vi "Markov Estimation.vi"(3 "UDP error in":errorcluster, 4 "UDP input cluster":T4, 5 "USRP error in":errorcluster, 6 "USRP input cluster":T3) -> (0 "ERROR":bool, 1 "UDP output cluster":T2, 2 "USRP output cluster":T1)   [LabVIEW 2014]
panel:
  out "Power":dbl[][](array[numeric])
  out "Delay":dbl[][](array[numeric])
  in  "Tab":enum32{"Interference", "Delay"}(tab)
  out "USRP error":errorcluster
  in  "Sampling Para.":T5={"Method"=enum."Binary", "offset"=0, "threshold"=1.0, "step"=1.0}
  in  "Number of Samplings":i32=100
  out "UDP error":errorcluster
  in  "Sampling Para2":T5
  in  "UDP parameter":T6={"remote IP Address"="192.168.1.101", "remote port"=54322, "local port(Tx)"=54321, "local port(Rx)"=54323}
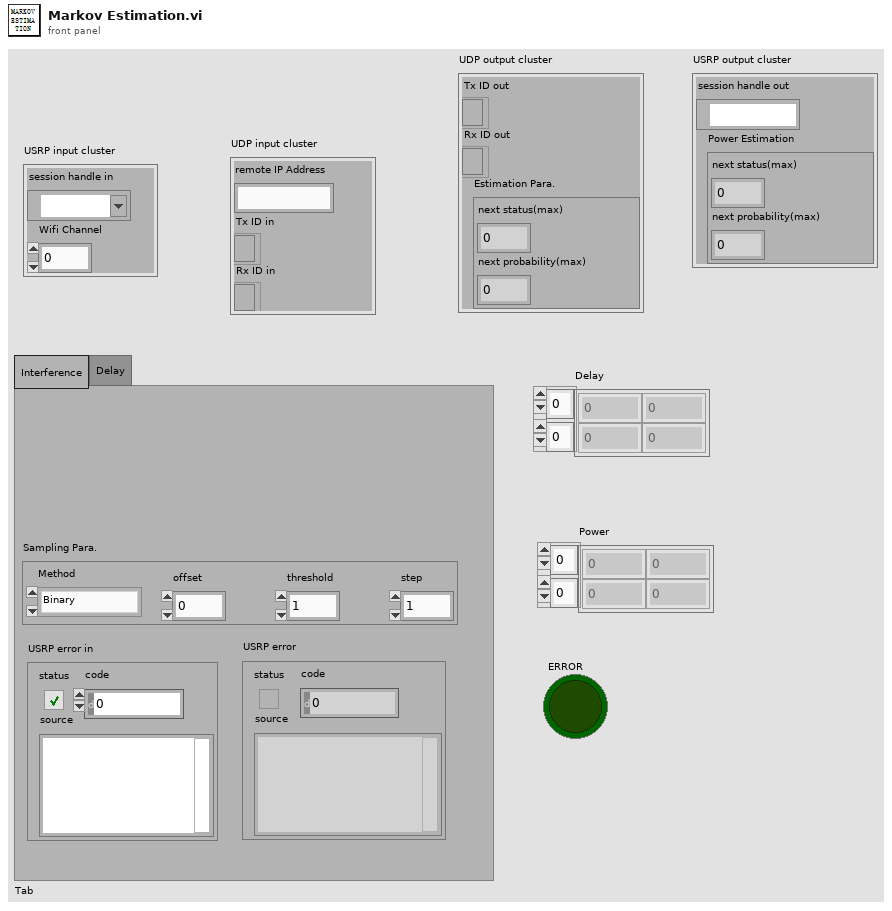
[diagram p1: front panel]
types:
  T1 = cluster{"session handle out":refnum<k15>, "Power Estimation":cluster{"next status(max)":i32, "next probability(max)":dbl}}
  T2 = cluster{"Tx ID out":refnum<k16>, "Rx ID out":refnum<k16>, "Estimation Para.":cluster{"next status(max)":i32, "next probability(max)":dbl}}
  T3 = cluster{"session handle in":refnum<k15>, "Wifi Channel":i32}
  T4 = cluster{"remote IP Address":string, "Tx ID in":refnum<k16>, "Rx ID in":refnum<k16>}
  T5 = cluster{"Method":enum16{"Binary", "Uniform"}, "offset":i32, "threshold":dbl, "step":dbl}
  T6 = cluster{"remote IP Address":string, "remote port":u16, "local port(Tx)":u16, "local port(Rx)":u16}
  T7 = cluster{"Tx ID out":refnum<k16>, "Rx ID out":refnum<k16>, "Delay Estimation":cluster{"next status(max)":i32, "next probability(max)":dbl}}
  T8 = cluster{"next status(max)":i32, "next probability(max)":dbl}
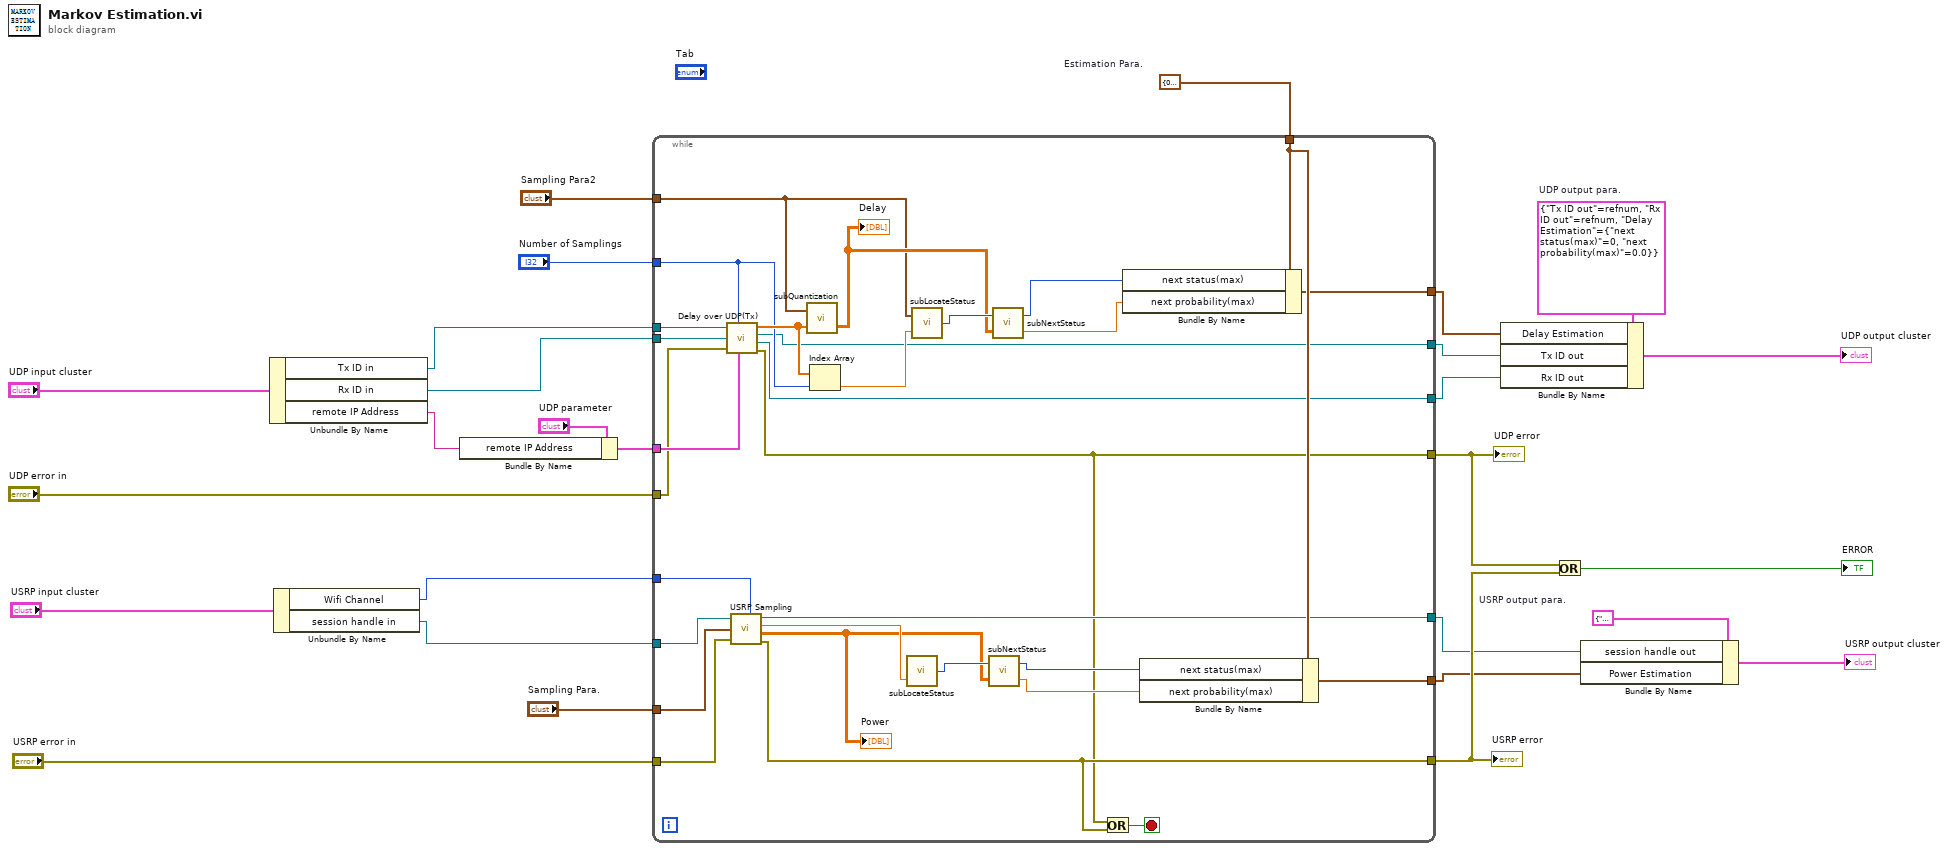
[diagram p0: block diagram]
diagram:
  w4 = T1 {"session handle out"="", "Power Estimation"={"next status(max)"=0, "next probability(max)"=0.0}}  # USRP output para.
  w9 = T7 {"Tx ID out"=refnum, "Rx ID out"=refnum, "Delay Estimation"={"next status(max)"=0, "next probability(max)"=0.0}}  # UDP output para.
  w24 = T8 {"next status(max)"=0, "next probability(max)"=0.0}  # Estimation Para.
  n1 = Unbundle By Name("UDP input cluster") -> ("Tx ID in"=w15:refnum<k16>, "Rx ID in"=w14:refnum<k16>, "remote IP Address"=w13:string)
  n2 = Unbundle By Name("USRP input cluster") -> ("Wifi Channel"=w11:i32, "session handle in"=w10:refnum<k15>)
  n3 = Bundle By Name(cluster="UDP parameter", "remote IP Address"=w13) -> (w17:T6)
  n4 = while {
    tunnel: [w56] -> w26
    tunnel: "Sampling Para2" -> [w50]
    tunnel: w24 -> [w49]
    tunnel: [w44] -> w8
    tunnel: [w43] -> w2
    tunnel: [w42] -> w3
    tunnel: "USRP error in" -> [w41]
    tunnel: w10 -> [w40]
    tunnel: "Sampling Para." -> [w39]
    tunnel: w11 -> [w38]
    tunnel: w17 -> [w37]
    tunnel: "UDP error in" -> [w36]
    tunnel: "Number of Samplings" -> [w33]
    tunnel: [w28] -> w19
    tunnel: w15 -> [w32]
    tunnel: w14 -> [w31]
    tunnel: [w30] -> w7
    tunnel: [w29] -> w6
    stop <- w57 stop-if-true
    n5 = call "Delay over UDP(Tx).vi"("Tx ID in"=w32, "Number of Samplings"=w33, "Rx ID in"=w31, "error in"=w36, "parameter"=w37) -> ("Output"=w35:dbl[], "Tx ID out"=w30:refnum<k16>, "Rx ID out"=w29:refnum<k16>, "error out"=w28:errorcluster)
    n6 = call "USRP Sampling.vi"("Wifi Channel"=w38, "error in"=w41, "parameter"=w39, "session handle in"=w40) -> ("error out"=w56:errorcluster, "output"=w51:dbl[][], "last value"=w52:dbl, "session handle out"=w42:refnum<k15>)
    "Power" <- w51
    n7 = call "subQuantization.vi"("input"=w35, "parameter"=w50) -> ("output"=w54:dbl[][])  [unwired: 1 out]
    "Delay" <- w54
    n8 = Index Array(array=w35, index=w33) -> (element=w34:dbl)
    n9 = call "subLocateStatus.vi"("Value"=w52) -> ("Status"=w53:i32)  [unwired: 1 in]
    n10 = call "subLocateStatus.vi"("Value"=w34, "parameter"=w50) -> ("Status"=w55:i32)
    n11 = call "subNextStatus.vi"("Markov Matrix"=w51, "Status"=w53) -> ("next probability(max)"=w45:dbl, "next status(max)"=w46:i32)
    n12 = call "subNextStatus.vi"("Markov Matrix"=w54, "Status"=w55) -> ("next probability(max)"=w47:dbl, "next status(max)"=w48:i32)
    n13 = Or(x=w28, y=w56) -> (x .or. y?=w57:bool)
    n14 = Bundle By Name(cluster=w49, "next status(max)"=w48, "next probability(max)"=w47) -> (w44:T8)
    n15 = Bundle By Name(cluster=w49, "next status(max)"=w46, "next probability(max)"=w45) -> (w43:T8)
  }
  "UDP error" <- w19
  "USRP error" <- w26
  n16 = Bundle By Name(cluster=w9, "Delay Estimation"=w8, "Tx ID out"=w7, "Rx ID out"=w6) -> (→"UDP output cluster":T7)
  n17 = Or(x=w19, y=w26) -> (x .or. y?=→"ERROR":bool)
  n18 = Bundle By Name(cluster=w4, "session handle out"=w3, "Power Estimation"=w2) -> (→"USRP output cluster":T1)
